vi "NumericToGameboard.vi"(8 "error in (no error)":errorcluster, 10 "CurrentPlayer":T1, 11 "NumericGameboard":i8[](array[numeric])) -> (0 "error out":errorcluster, 3 "Gameboard":T2)   [LabVIEW 2020]
uses:
  controls/Gameboard Data.ctl
  controls/Player.ctl
  <vilib>/Utility/error.llb/Error Cluster From Error Code.vi
  <vilib>/ErrorRing/Error Ring.xnode
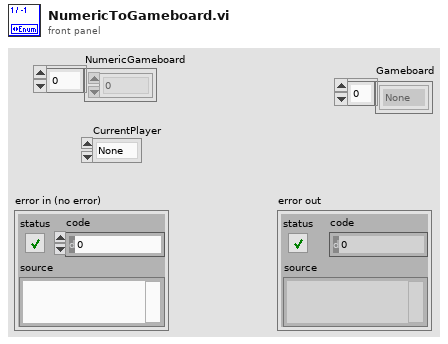
[diagram p1: front panel]
types:
  T1 = typedef "Player.ctl" = enum16{"None", "Player 1", "Player 2"}
  T2 = typedef "Gameboard Data.ctl" = enum16{"None", "Player 1", "Player 2"}[]
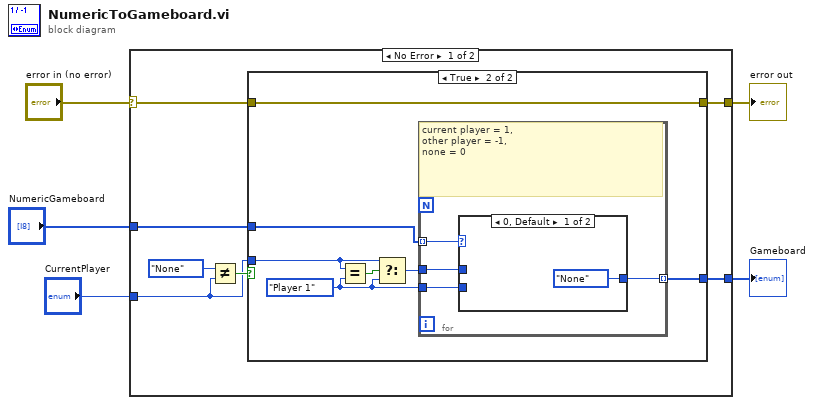
[diagram p0: block diagram]
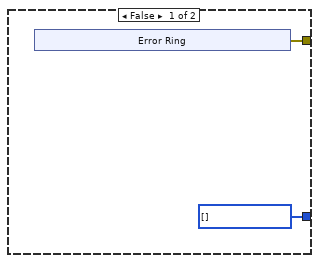
[diagram p2: hidden frame]
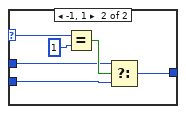
[diagram p3: hidden frame]
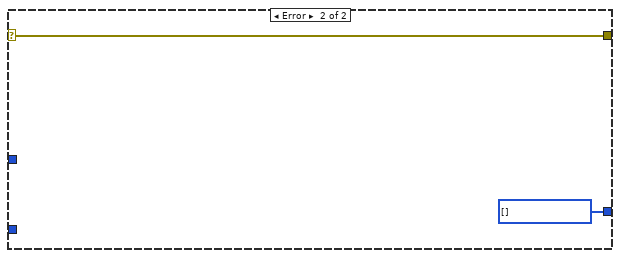
[diagram p4: hidden frame]
diagram:
  n1 = case shown="No Error" "error in (no error)" {
    selector: "error in (no error)" -> [w7 w38]
    tunnel: [w12 w39] -> w5
    tunnel: "NumericGameboard" -> [w10 _]
    tunnel: "CurrentPlayer" -> [w9 _]
    tunnel: [w6 w38] -> w1
    frame No Error {
      n2 = Not Equal?(x=Player."None", y=w9) -> (x != y?=w11:bool)
      n3 = case shown="True" w11 {
        tunnel: w10 -> [_ w26]
        tunnel: w9 -> [_ w24]
        tunnel: [w14 w22] -> w12
        tunnel: w7 -> [_ w20]
        tunnel: [w13 w20] -> w6
        frame False {
          w14 = T1[] [] items=["None", "Player 1", "Player 2"]
          n4 = xnode "Error Ring"() -> ("error out"=w13:errorcluster)
        }
        frame True {
          w21 = Player."Player 1" ("y")
          n5 = Equal?(x=w24, y=w21) -> (x = y?=w23:bool)
          n6 = Select(t=w24, s=w23, f=w21) -> (s? t:f=w25:T1)
          n7 = for {
            tunnel: w26 -> [w30] mode=indexing
            tunnel: w25 -> [w29]
            tunnel: [w28] -> w22 mode=indexing
            tunnel: w21 -> [w27]
            # "current player = 1,\nother player = -1,\nnone = 0"
            n8 = case shown="0, Default" w30 {
              selector: w30 -> [_ w37]
              tunnel: w29 -> [_ w33]
              tunnel: [Player."None" ("y") w35] -> w28
              tunnel: w27 -> [_ w32]
              frame 0, Default {
              }
              frame -1, 1 {
                n9 = Equal?(x=w37, y=i8 1) -> (x = y?=w36:bool)
                n10 = Select(t=w33, s=w36, f=w32) -> (s? t:f=w35:T1)
              }
            }
          }
        }
      }
    }
    frame Error {
      w39 = T1[] [] items=["None", "Player 1", "Player 2"]
    }
  }
  "Gameboard" <- w5
  "error out" <- w1
